vi "Play Path.vi"(7 "Description":string, 8 "Command Info In":T2, 11 "Auto Velocities":T1[](array[typedef])) -> (0 "Command Info Out":T2)   [LabVIEW 2020]
doc: "This VI notifies the subsystem to the new setpoint."
uses:
  <vilib>/Rock Robotics/WPI/Framework/Command Status Info.ctl
  <vilib>/Rock Robotics/WPI/Framework/Completion Status.ctl
  <vilib>/Rock Robotics/WPI/Framework/Completion Notifier.ctl
  Implementation/Robot Velocities.ctl
  Implementation/Drive Setpoints.ctl
  Implementation/Drive Operations.ctl
  <vilib>/Rock Robotics/WPI/ThirdParty/Phoenix-LabVIEW/Motor Controller/Controls/CTRE_Phoenix_MotorControl_ControlMode.ctl
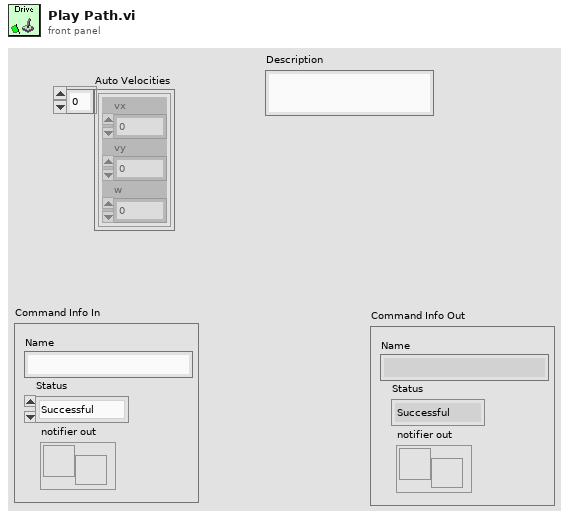
[diagram p1: front panel]
types:
  T1 = typedef "Robot Velocities.ctl" = cluster{"vx":dbl, "vy":dbl, "w":dbl}
  T2 = typedef "Command Status Info.ctl" = cluster{"Name":string, "Status":T3, "notifier out":T4}
  T3 = typedef "Completion Status.ctl" = enum16{"Successful", "Aborted", "Incomplete"}
  T4 = typedef "Completion Notifier.ctl" = refnum<notifier>
  T5 = typedef "Drive Setpoints.ctl" = cluster{"Operation":T6, "Robot Velocities":T1, "Field Centric?":bool, "Auto Velocities":T1[], "Manual Parameters":cluster{"Control Mode":T7, "Motor Type":enum16{"Drive", "Steer"}, "Control Units":enum16{"Raw Units", "Rotations", "Real Units"}, "Setpoints":cluster{"Left Front":dbl, "Left Back":dbl, "Right Front":dbl, "Right Back":dbl}, "Time Delay":dbl}}
  T6 = typedef "Drive Operations.ctl" = enum16{"Reserve", "Read Current", "Immediate", "Calibrate", "Reset Pods", "Auto", "Manual Pod Debugging"}
  T7 = typedef "CTRE_Phoenix_MotorControl_ControlMode.ctl" = u16
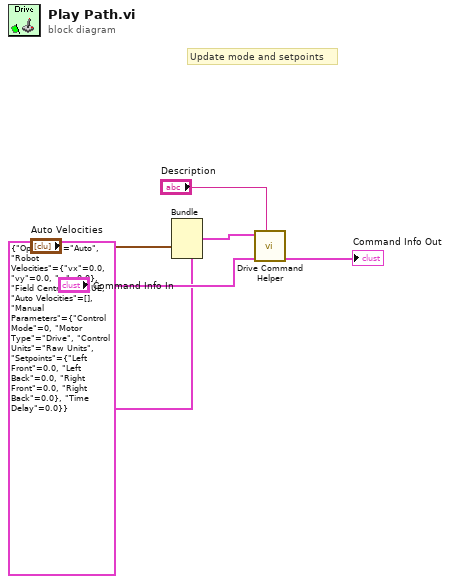
[diagram p0: block diagram]
diagram:
  # "Update mode and setpoints"
  n1 = Bundle(cluster=T5 {"Operation"=enum."Auto", "Robot Velocities"={"vx"=0.0, "vy"=0.0, "w"=0.0}, "Field Centric?"=TRUE, "Auto Velocities"=[], "Manual Parameters"={"Control Mode"=0, "Motor Type"=enum."Drive", "Control Units"=enum."Raw Units", "Setpoints"={"Left Front"=0.0, "Left Back"=0.0, "Right Front"=0.0, "Right Back"=0.0}, "Time Delay"=0.0}} ("SubSystem Data"), "Auto Velocities"="Auto Velocities") -> (w3:T5)  [unwired: 4 in]
  n2 = call "Drive Command Helper.vi"("Description"="Description", "Command Info In"="Command Info In", "SubSystem Data"=w3) -> ("Command Info Out"=→"Command Info Out":T2)  [unwired: 6 in, 2 out]
